vi "Der_A.vi"(1 "dZ_l":T1, 2 "W_l":T1) -> (0 "dA_l-1":T1)   [LabVIEW 2016]
uses:
  <vilib>/Analysis/Matrix/Datatypes/RealMatrix.ctl
  <vilib>/Analysis/Matrix/Numeric/Multiply/Multiply - RM,RM.vi
  <vilib>/Analysis/Matrix/NI_Matrix.lvlib
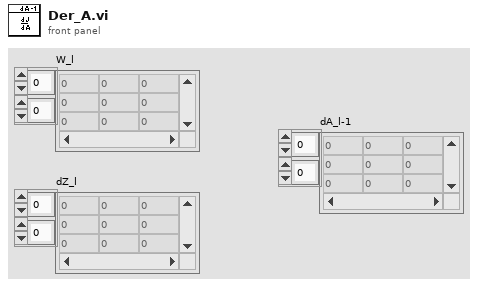
[diagram p1: front panel]
types:
  T1 = typedef "NI_Matrix.lvlib/RealMatrix.ctl" = dbl[][]
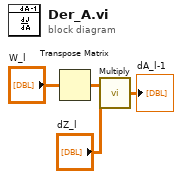
[diagram p0: block diagram]
diagram:
  n1 = Transpose Matrix(1:"W_l") -> (0:w3:T1)
  n2 = call-poly <vilib>:"Multiply.vi"("Real Matrix B"="dZ_l", "Real Matrix A"=w3) -> ("A * B"=→"dA_l-1":T1)
